vi "Limit Switch.vi"() -> ()   [LabVIEW 2014]
uses:
  <vilib>/Rock Robotics/SystemInterfaces/DIO/FPGA_DIOChannel.ctl
  <vilib>/Rock Robotics/SystemInterfaces/AI/FPGA_AIChannel.ctl
panel:
  out "Voltage":dbl
  out "Value 3":bool
  out "Value 2":bool
  out "Value":bool
  out "Boolean":bool
  in  "Mode":enum8{"Start", "Run", "Finish"}(ring)
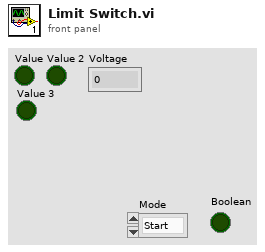
[diagram p1: front panel]
types:
  T1 = typedef "FPGA_AIChannel.ctl" = enum8{"AI 0", "AI 1", "AI 2", "AI 3", "AI MXP 0", "AI MXP 1", "AI MXP 2", "AI MXP 3", "Invalid"}
  T2 = typedef "FPGA_DIOChannel.ctl" = enum8{"DIO 0", "DIO 1", "DIO 2", "DIO 3", "DIO 4", "DIO 5", "DIO 6", "DIO 7", "DIO 8", "DIO 9", "DIO MXP 0", "DIO MXP 1", "DIO MXP 2", "DIO MXP 3", "DIO MXP 4", "DIO MXP 5", "DIO MXP 6", "DIO MXP 7", "DIO MXP 8", "DIO MXP 9", "DIO MXP 10", "DIO MXP 11", "DIO MXP 12", "DIO MXP 13", "DIO MXP 14", "DIO MXP 15", "Invalid"}
  T3 = typedef "WPI_DigitalInputDevRef.ctl" = cluster{"DevStatus":errorcluster, "DIO Channel":T2, "Controller":T4}
  T4 = typedef "FPGA_TypedefDigitalModule.ctl" = enum16{"Controller 1"}
  T5 = typedef "WPI_AnalogChannelDevRef.ctl" = cluster{"DevStatus":errorcluster, "Controller":T6, "Analog Channel":T1}
  T6 = typedef "FPGA_TypedefAnalogModule.ctl" = enum16{"Controller 1"}
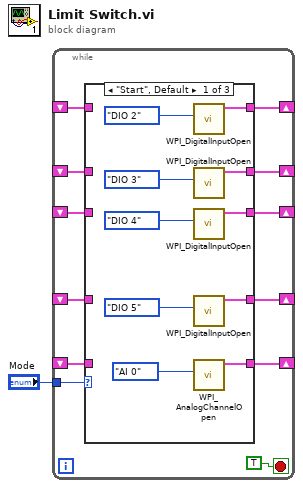
[diagram p0: block diagram]
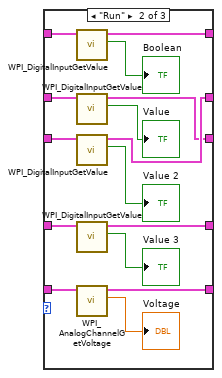
[diagram p2: hidden frame]
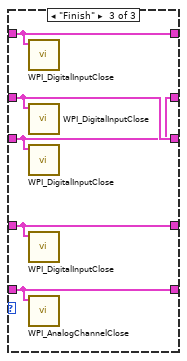
[diagram p3: hidden frame]
diagram:
  n1 = while {
    tunnel: "Mode" -> [w13]
    shift-right: [w12] -> _
    shift-left: _ -> [w11]
    shift-right: [w9] -> _
    shift-left: _ -> [w5]
    shift-right: [w8] -> _
    shift-left: _ -> [w4]
    shift-right: [w7] -> _
    shift-left: _ -> [w3]
    shift-right: [w6] -> _
    shift-left: _ -> [w2]
    stop <- TRUE stop-if-true
    n2 = case shown="\"Start\", Default" w13 {
      tunnel: [w22 w37 w43] -> w12
      tunnel: w11 -> [_ w38 w43]
      tunnel: [w17 w25 w39] -> w9
      tunnel: [w16 w24 w41] -> w8
      tunnel: [w15 w26 w40] -> w7
      tunnel: [w14 w28 w42] -> w6
      tunnel: w5 -> [_ w35 w41]
      tunnel: w4 -> [_ w34 w39]
      tunnel: w3 -> [_ w33 w40]
      tunnel: w2 -> [_ w29 w42]
      frame "Start", Default {
        n3 = call <vilib>:"WPI_DigitalInputOpen.vi"("DIO Channel"=FPGA_DIOChannel."DIO 2") -> ("DigitalInputDevRef"=w22:T3)  [unwired: 9 in, 1 out]
        n4 = call <vilib>:"WPI_DigitalInputOpen.vi"("DIO Channel"=FPGA_DIOChannel."DIO 3") -> ("DigitalInputDevRef"=w17:T3)  [unwired: 9 in, 1 out]
        n5 = call <vilib>:"WPI_DigitalInputOpen.vi"("DIO Channel"=FPGA_DIOChannel."DIO 4") -> ("DigitalInputDevRef"=w16:T3)  [unwired: 9 in, 1 out]
        n6 = call <vilib>:"WPI_DigitalInputOpen.vi"("DIO Channel"=FPGA_DIOChannel."DIO 5") -> ("DigitalInputDevRef"=w15:T3)  [unwired: 9 in, 1 out]
        n7 = call <vilib>:"WPI_AnalogChannelOpen.vi"("Analog Channel"=FPGA_AIChannel."AI 0") -> ("AIDeviceRef"=w14:T5)  [unwired: 9 in, 1 out]
      }
      frame "Run" {
        n8 = call <vilib>:"WPI_DigitalInputGetValue.vi"("DigitalInputDevRef"=w38) -> ("Value"=→"Boolean":bool, "DigitalInputDevRef"=w37:T3)  [unwired: 8 in, 1 out]
        n9 = call <vilib>:"WPI_DigitalInputGetValue.vi"("DigitalInputDevRef"=w35) -> ("Value"=→"Value":bool, "DigitalInputDevRef"=w24:T3)  [unwired: 8 in, 1 out]
        n10 = call <vilib>:"WPI_DigitalInputGetValue.vi"("DigitalInputDevRef"=w34) -> ("Value"=→"Value 2":bool, "DigitalInputDevRef"=w25:T3)  [unwired: 8 in, 1 out]
        n11 = call <vilib>:"WPI_DigitalInputGetValue.vi"("DigitalInputDevRef"=w33) -> ("Value"=→"Value 3":bool, "DigitalInputDevRef"=w26:T3)  [unwired: 8 in, 1 out]
        n12 = call <vilib>:"WPI_AnalogChannelGetVoltage.vi"("AIDeviceRef"=w29) -> ("Voltage"=→"Voltage":dbl, "AIDeviceRef"=w28:T5)  [unwired: 8 in, 1 out]
      }
      frame "Finish" {
        n13 = call <vilib>:"WPI_DigitalInputClose.vi"("DigitalInputDevRef"=w43) -> ()  [unwired: 10 in, 1 out]
        n14 = call <vilib>:"WPI_DigitalInputClose.vi"("DigitalInputDevRef"=w41) -> ()  [unwired: 10 in, 1 out]
        n15 = call <vilib>:"WPI_DigitalInputClose.vi"("DigitalInputDevRef"=w39) -> ()  [unwired: 10 in, 1 out]
        n16 = call <vilib>:"WPI_DigitalInputClose.vi"("DigitalInputDevRef"=w40) -> ()  [unwired: 10 in, 1 out]
        n17 = call <vilib>:"WPI_AnalogChannelClose.vi"("AIDeviceRef"=w42) -> ()  [unwired: 10 in, 1 out]
      }
    }
  }
